vi "Try Auto Connect.vi"(7 "Main VI":refnum<vi>, 8 "Error In":errorcluster, 11 "Connection Status":T1) -> (0 "Error Out":errorcluster, 3 "Connection Status Out":T1, 4 "VISA resource name OUT":refnum<visa-resource-name>)   [LabVIEW 2014]
doc: "This VI tries to automatically find and connect The Reaper"
uses:
  Controls/Connection Status.ctl
panel:
  in  "No Button":bool
  in  "Yes Button":bool
  # "It may take a while. Do you want to continue?"
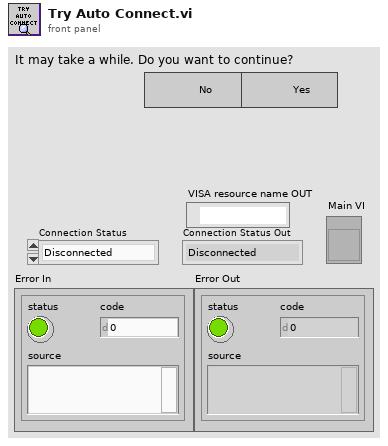
[diagram p1: front panel]
types:
  T1 = typedef "Connection Status.ctl" = enum16{"Disconnected", "Connected"}
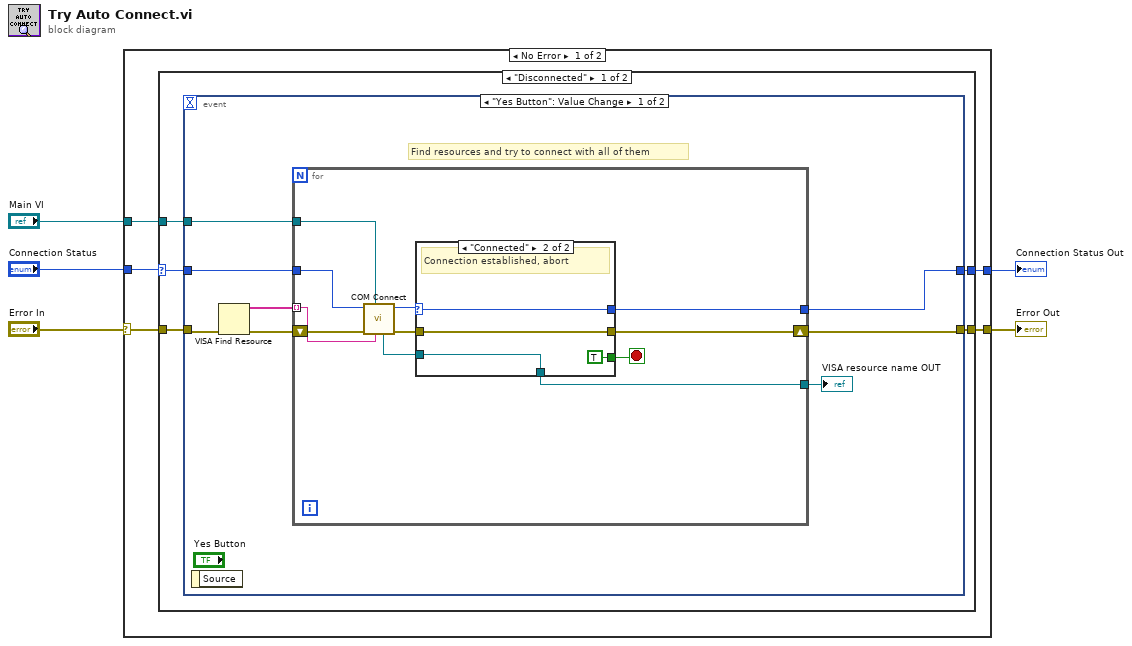
[diagram p0: block diagram]
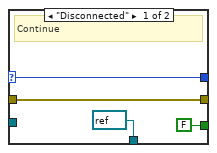
[diagram p2: hidden frame]
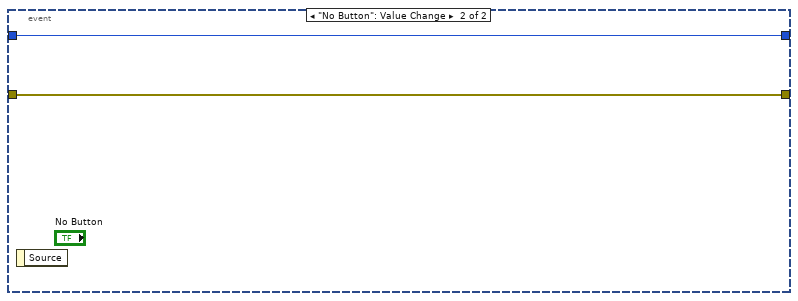
[diagram p3: hidden frame]
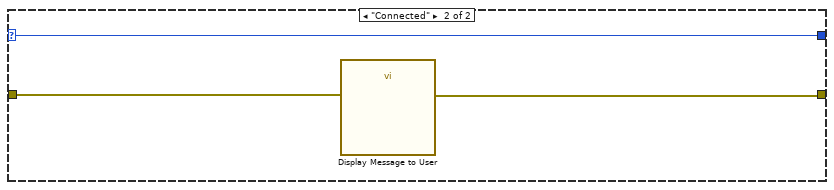
[diagram p4: hidden frame]
diagram:
  n1 = case shown="No Error" "Error In" {
    selector: "Error In" -> [w8 w48]
    tunnel: "Connection Status" -> [w10 w49]
    tunnel: [w9 w49] -> w3
    tunnel: [w7 w48] -> w2
    tunnel: "Main VI" -> [w6 _]
    frame No Error {
      n2 = case shown="\"Disconnected\"" w10 {
        selector: w10 -> [w13 w47]
        tunnel: [w12 w47] -> w9
        tunnel: w8 -> [w15 w46]
        tunnel: [w14 w45] -> w7
        tunnel: w6 -> [w11 _]
        frame "Disconnected" {
          n3 = event shown="[0] \"Yes Button\": Value Change" {
            selector: _ -> [_ _]
            dyn-events: _ -> [_ _]
            timeout: _ -> [_ _]
            tunnel: w15 -> [w23 w44]
            tunnel: [w18 w44] -> w14
            tunnel: w13 -> [w21 w43]
            tunnel: [w17 w43] -> w12
            tunnel: w11 -> [w19 _]
            event "Yes Button": Value Change {
              # "Find resources and try to connect with all of them"
              n4 = event-data() -> ()  [unwired: 1 in, 1 out]
              n5 = VISA Find Resource(8:w23) -> (0:w20:errorcluster, 3:w22:string[])  [unwired: 2 in, 1 out]
              n6 = for {
                tunnel: w22 -> [w32] mode=indexing
                tunnel: w21 -> [w33]
                shift-right: [w27] -> w18
                shift-left: w20 -> [w34]
                tunnel: w19 -> [w29]
                tunnel: [w26] -> w17
                tunnel: [w24] -> w16
                stop <- w28 stop-if-true
                n7 = call "COM Connect.vi"("VISA resource name"=w32, "Main Front Panel Ref"=w29, "Error In"=w34, "Connection Status"=w33) -> ("Error Out"=w30:errorcluster, "Connection Status"=w31:T1, "VISA resource name OUT"=w25:refnum<visa-resource-name>)  [unwired: 5 in]
                n8 = case shown="\"Connected\"" w31 {
                  selector: w31 -> [w36 w40]
                  tunnel: w30 -> [w37 w41]
                  tunnel: [FALSE TRUE] -> w28
                  tunnel: [w37 w41] -> w27
                  tunnel: [w36 w40] -> w26
                  tunnel: w25 -> [_ w39]
                  tunnel: [refnum<visa-resource-name> refnum ("VISA resource name OUT") w39] -> w24
                  frame "Disconnected" {
                    # "Continue"
                  }
                  frame "Connected" {
                    # "Connection established, abort"
                  }
                }
              }
              "VISA resource name OUT" <- w16
            }
            event "No Button": Value Change {
              n9 = event-data() -> ()  [unwired: 1 in, 1 out]
            }
          }
        }
        frame "Connected" {
          n10 = call "Display Message to User"("error in (no error)"=w46) -> ("error out"=w45:errorcluster)  [unwired: 9 in, 1 out]
        }
      }
    }
    frame Error {
    }
  }
  "Error Out" <- w2
  "Connection Status Out" <- w3
